vi "DEPLOY THIS VI REPORT FRONT PANEL WRITE IMAGE.vi"() -> ()   [LabVIEW 2013]
panel:
  out "path":path=path "D:/FINALE @25 #bangalore/IMG-20170928-WA0001 - Copy"
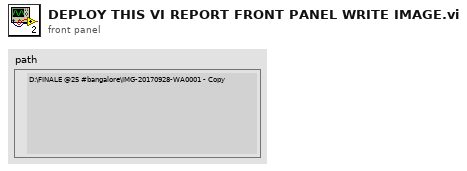
[diagram p1: front panel]
types:
  T1 = typedef "imagedata.ctl" = cluster{"image type":i32, "image depth":i32, "image":u8[], "mask":u8[], "colors":u32[], "Rectangle":cluster{"left":i16, "top":i16, "right":i16, "bottom":i16}}
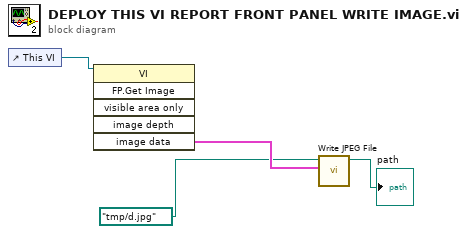
[diagram p0: block diagram]
diagram:
  n1 = control-ref of="This VI"() -> (w3:refnum<vi>)
  n2 = invoke class="VI" method="FP.Get Image"(reference=w3) -> ("image data"=w4:T1)  [unwired: 5 in, 5 out]
  n3 = call <vilib>:"Write JPEG File.vi"("image data"=w4, "path to JPEG file"=path "/tmp/d.jpg") -> ("path"=→"path":path)  [unwired: 8 in, 1 out]
